vi "lab3_xyzp_nand.vi"() -> ()   [LabVIEW 2023]
panel:
  out "y":bool
  in  "p_in":bool
  in  "z_in":bool
  in  "y_in":bool
  in  "x_in":bool
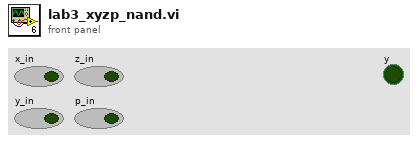
[diagram p1: front panel]
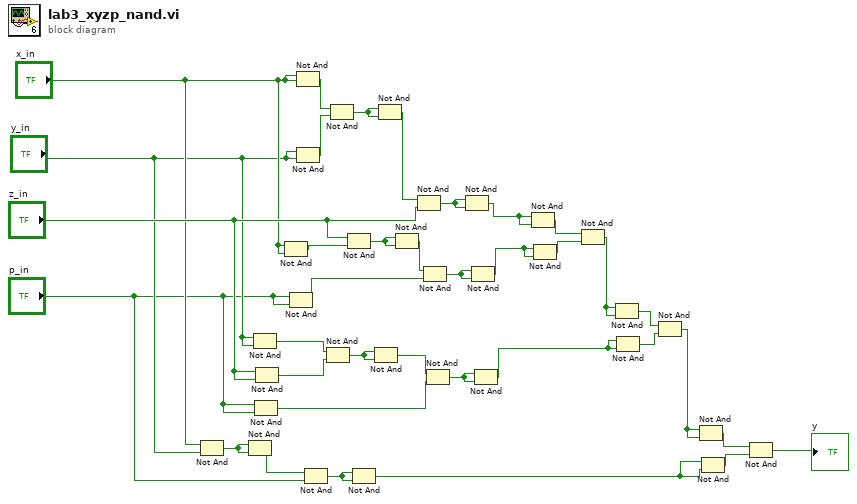
[diagram p0: block diagram]
diagram:
  n1 = Not And(1:"y_in", 2:"x_in") -> (0:w9:bool)
  n2 = Not And(1:w9, 2:w9) -> (0:w5:bool)
  n3 = Not And(1:"y_in", 2:"y_in") -> (0:w24:bool)
  n4 = Not And(1:"p_in", 2:"p_in") -> (0:w20:bool)
  n5 = Not And(1:"z_in", 2:"z_in") -> (0:w23:bool)
  n6 = Not And(1:"x_in", 2:"x_in") -> (0:w30:bool)
  n7 = Not And(1:"p_in", 2:"p_in") -> (0:w27:bool)
  n8 = Not And(1:"x_in", 2:"x_in") -> (0:w35:bool)
  n9 = Not And(1:"y_in", 2:"y_in") -> (0:w34:bool)
  n10 = Not And(1:"p_in", 2:w5) -> (0:w6:bool)
  n11 = Not And(1:w23, 2:w24) -> (0:w25:bool)
  n12 = Not And(1:w34, 2:w35) -> (0:w36:bool)
  n13 = Not And(1:w30, 2:"z_in") -> (0:w31:bool)
  n14 = Not And(1:w6, 2:w6) -> (0:w3:bool)
  n15 = Not And(1:w25, 2:w25) -> (0:w21:bool)
  n16 = Not And(1:w36, 2:w36) -> (0:w32:bool)
  n17 = Not And(1:w31, 2:w31) -> (0:w28:bool)
  n18 = Not And(1:"z_in", 2:w32) -> (0:w33:bool)
  n19 = Not And(1:w27, 2:w28) -> (0:w29:bool)
  n20 = Not And(1:w20, 2:w21) -> (0:w22:bool)
  n21 = Not And(1:w33, 2:w33) -> (0:w19:bool)
  n22 = Not And(1:w29, 2:w29) -> (0:w18:bool)
  n23 = Not And(1:w22, 2:w22) -> (0:w12:bool)
  n24 = Not And(1:w19, 2:w19) -> (0:w16:bool)
  n25 = Not And(1:w18, 2:w18) -> (0:w17:bool)
  n26 = Not And(1:w17, 2:w16) -> (0:w13:bool)
  n27 = Not And(1:w13, 2:w13) -> (0:w14:bool)
  n28 = Not And(1:w12, 2:w12) -> (0:w15:bool)
  n29 = Not And(1:w15, 2:w14) -> (0:w2:bool)
  n30 = Not And(1:w2, 2:w2) -> (0:w10:bool)
  n31 = Not And(1:w3, 2:w3) -> (0:w11:bool)
  n32 = Not And(1:w11, 2:w10) -> (0:→"y":bool)
